vi "Image_Line_evaluation.vi"(11 "RawImageData":u16[](array[numeric])) -> (3 "Error":dbl)   [LabVIEW 2020]
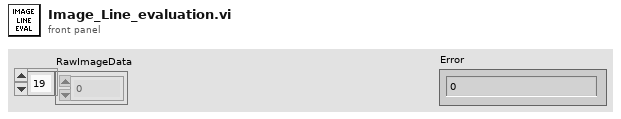
[diagram p1: front panel]
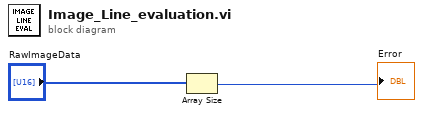
[diagram p0: block diagram]
diagram:
  n1 = Array Size(array="RawImageData") -> (size(s)=→"Error":i32)
